vi "Free_dynamics_test.vi"() -> ()   [LabVIEW 2018]
uses:
  <vilib>/Analysis/coordinate.llb/Euler Rotation Order.ctl
  <vilib>/imath/engines/lvmath2/RunTimeEngine/NodeEndStatement/NIMS_NodeEndStatement_Output.vi
  <instcachedir>/0/NIMS_NodeEndStatement_Output_53EC0D466D134D7ABD903AC30B43404B.lvgen/NIMS_NodeEndStatement_Output_53EC0D466D134D7ABD903AC30B43404B_009.vi
  <vilib>/imath/engines/lvmath2/RunTimeEngine/ErrorHandling/NIMS_Finalize Error.vi
  <instcachedir>/0/NIMS_NodeEndStatement_Output_53EC0D466D134D7ABD903AC30B43404B.lvgen/NIMS_NodeEndStatement_Output_53EC0D466D134D7ABD903AC30B43404B_004.vi
  <vilib>/Analysis/baseanly.llb/Real Inverse Matrix.vi
  <vilib>/Analysis/Matrix/Numeric/Conversions/Array To Matrix - RA.vi
  <vilib>/Analysis/Matrix/Numeric/Conversions/Matrix To Array - RM.vi
  <vilib>/imath/engines/lvmath2/RunTimeEngine/IndexRead/NIMS M(S).vi
  <instcachedir>/0/NIMS M(S)_B826C018497E4940AE96BD27B540B6FB.lvgen/NIMS M(S)_B826C018497E4940AE96BD27B540B6FB_000.vi
  <vilib>/imathl/engines/lvmath/Functions/Error Handling/Create Error.vi
  <vilib>/imath/engines/lvmath2/RunTimeEngine/IndexRead/NIMS V(S).vi
  <instcachedir>/0/NIMS V(S)_0488751826AF41519A22953C041130DC.lvgen/NIMS V(S)_0488751826AF41519A22953C041130DC_000.vi
  <vilib>/imath/engines/lvmath2/RunTimeEngine/BuiltInFunctions/cross/NIMS_cross(GV,GV).vi
  <instcachedir>/0/NIMS_cross(GV,GV)_8E551EB9DC304C30866B49598818C259.lvgen/NIMS_cross(GV,GV)_8E551EB9DC304C30866B49598818C259_000.vi
  <vilib>/imath/engines/lvmath2/RunTimeEngine/BuiltInFunctions/double/NIMS_double.vi
  <instcachedir>/0/NIMS_double_34E32F64C2B04A25A042F4CA881A0A41.lvgen/NIMS_double_34E32F64C2B04A25A042F4CA881A0A41_002.vi
  <vilib>/imath/engines/lvmath2/RunTimeEngine/ArithmeticOperatorToken/NIMS_ArithmeticOperator_multmx.vi
  <instcachedir>/0/NIMS_ArithmeticOperator_multmx_622CA76F9646436AB036D42A9A1CE0E6.lvgen/NIMS_ArithmeticOperator_multmx_622CA76F9646436AB036D42A9A1CE0E6_004.vi
  <vilib>/imath/engines/lvmath2/RunTimeEngine/BuiltInFunctions/cross/NIMS_cross(GM,GM,I32).vi
  <instcachedir>/0/NIMS_cross(GM,GM,I32)_0F6D45CF7D834A0BB6695B819A7F63BC.lvgen/NIMS_cross(GM,GM,I32)_0F6D45CF7D834A0BB6695B819A7F63BC_000.vi
  <vilib>/imath/engines/lvmath2/RunTimeEngine/ArithmeticOperatorToken/NIMS_ArithmeticOperator_plus.vi
  <instcachedir>/0/NIMS_ArithmeticOperator_plus_DE670E32103C4C10ADF2A97367172B30.lvgen/NIMS_ArithmeticOperator_plus_DE670E32103C4C10ADF2A97367172B30_003.vi
  <vilib>/imath/engines/lvmath2/RunTimeEngine/ErrorHandling/NIMS_Create Error From Enums.vi
  <instcachedir>/0/NIMS_double_34E32F64C2B04A25A042F4CA881A0A41.lvgen/NIMS_double_34E32F64C2B04A25A042F4CA881A0A41_003.vi
  <vilib>/imath/engines/lvmath2/RunTimeEngine/ArithmeticOperatorToken/NIMS_ArithmeticOperator_multmx-internal.vi
  <instcachedir>/0/NIMS_ArithmeticOperator_multmx-internal_16A6E1DA326644AB974D30232E729C42.lvgen/NIMS_ArithmeticOperator_multmx-internal_16A6E1DA326644AB974D30232E729C42_004.vi
  <vilib>/imath/engines/lvmath2/RunTimeEngine/NodeEndStatement/NIMS_NodeEndStatement_Get Vector.vi
  <instcachedir>/0/NIMS_NodeEndStatement_Get Vector_329D0992E87F49F089135171B7FC9327.lvgen/NIMS_NodeEndStatement_Get Vector_329D0992E87F49F089135171B7FC9327_001.vi
  <vilib>/imath/engines/lvmath/Functions/Error Handling/MergeErrorsWrapper.vi
  <instcachedir>/0/NIMS_NodeEndStatement_Output_53EC0D466D134D7ABD903AC30B43404B.lvgen/NIMS_NodeEndStatement_Output_53EC0D466D134D7ABD903AC30B43404B_002.vi
  <instcachedir>/0/NIMS_NodeEndStatement_Output_53EC0D466D134D7ABD903AC30B43404B.lvgen/NIMS_NodeEndStatement_Output_53EC0D466D134D7ABD903AC30B43404B_005.vi
  <vilib>/Analysis/NI_AALPro.lvlib
  <vilib>/Analysis/Matrix/NI_Matrix.lvlib
  <vilib>/Analysis/NI_AALBase.lvlib
panel:
  out "W":dbl[](array[numeric])
  out "Yaw 2":dbl(graph)
  out "Pitch 2":dbl(graph)
  out "Roll 2":dbl(graph)
  out "Attitude 2":cluster{"phi":dbl, "theta":dbl, "psi":dbl}
  in  "Mass (kg)":dbl
  in  "MOI(kg*m^2)":dbl[][](array[numeric])
  in  "COG(m)":dbl[](array[numeric])
  in  "Simulation Time(sec)":dbl
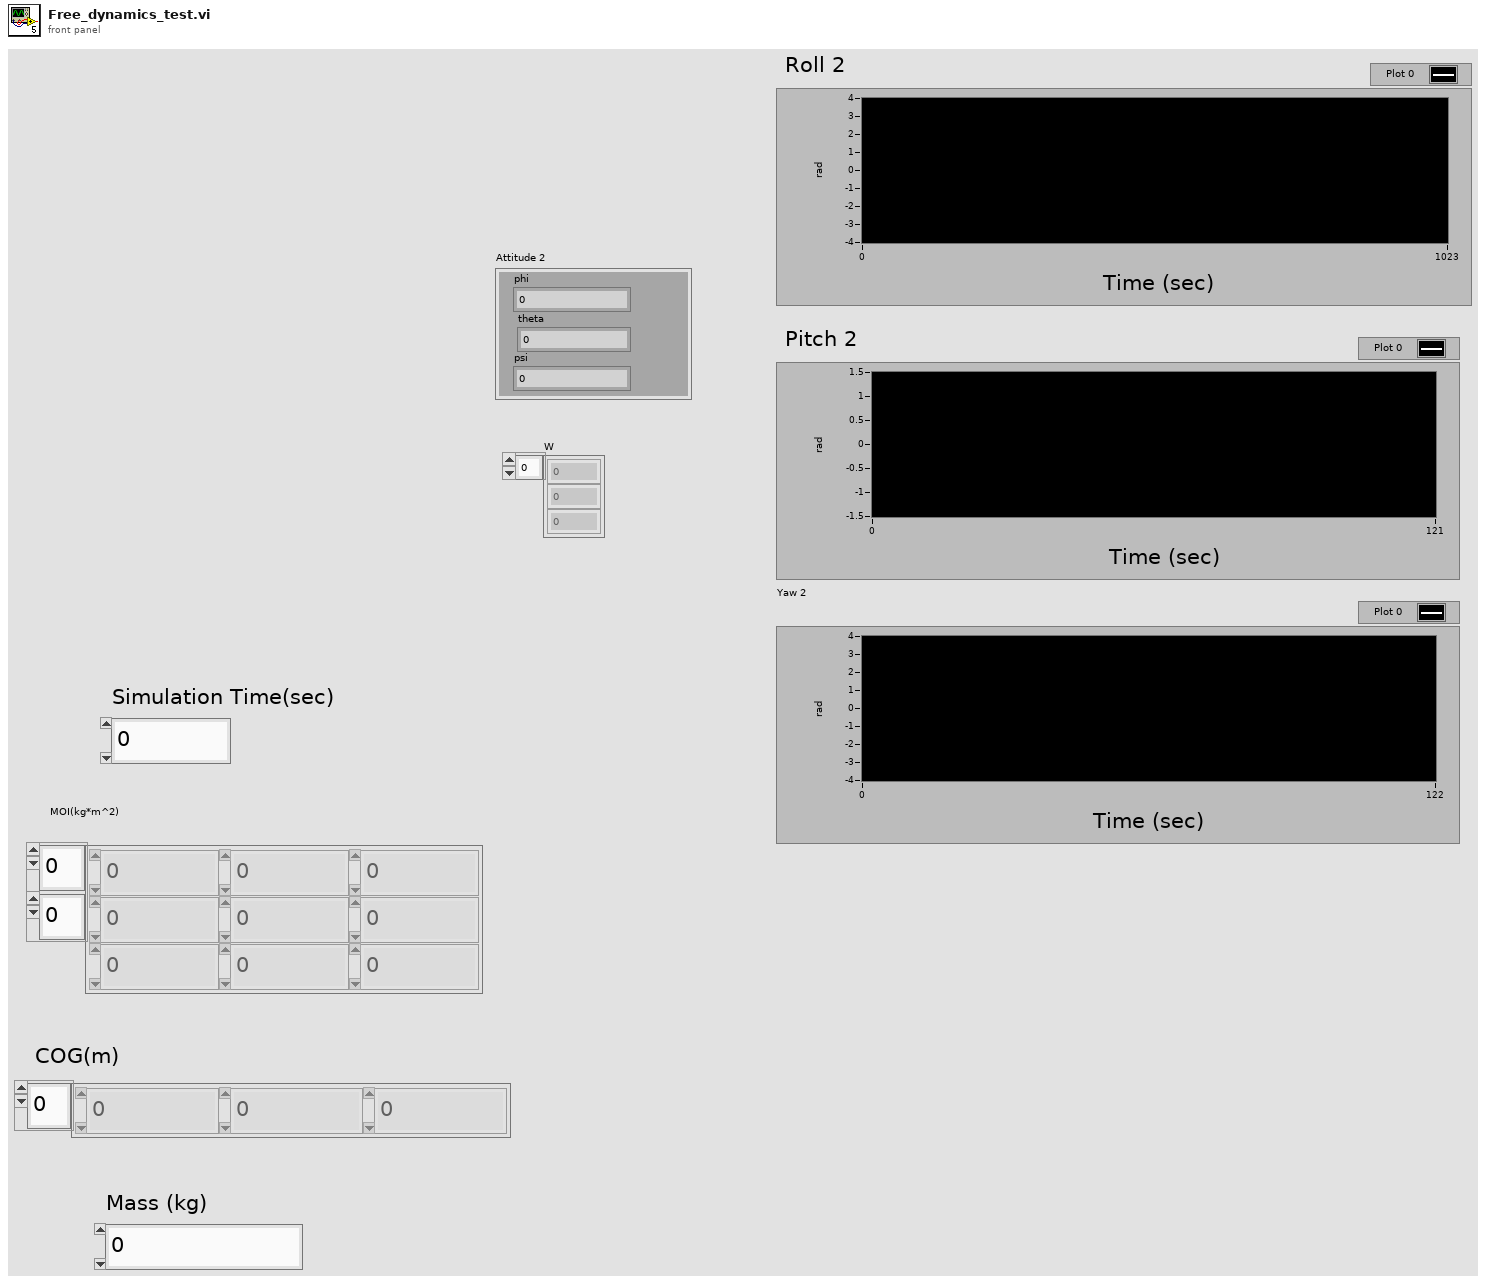
[diagram p1: front panel]
types:
  T1 = typedef "NI_AALPro.lvlib/Euler Rotation Order.ctl" = u16
  T2 = typedef "NI_Matrix.lvlib/RealMatrix.ctl" = dbl[][]
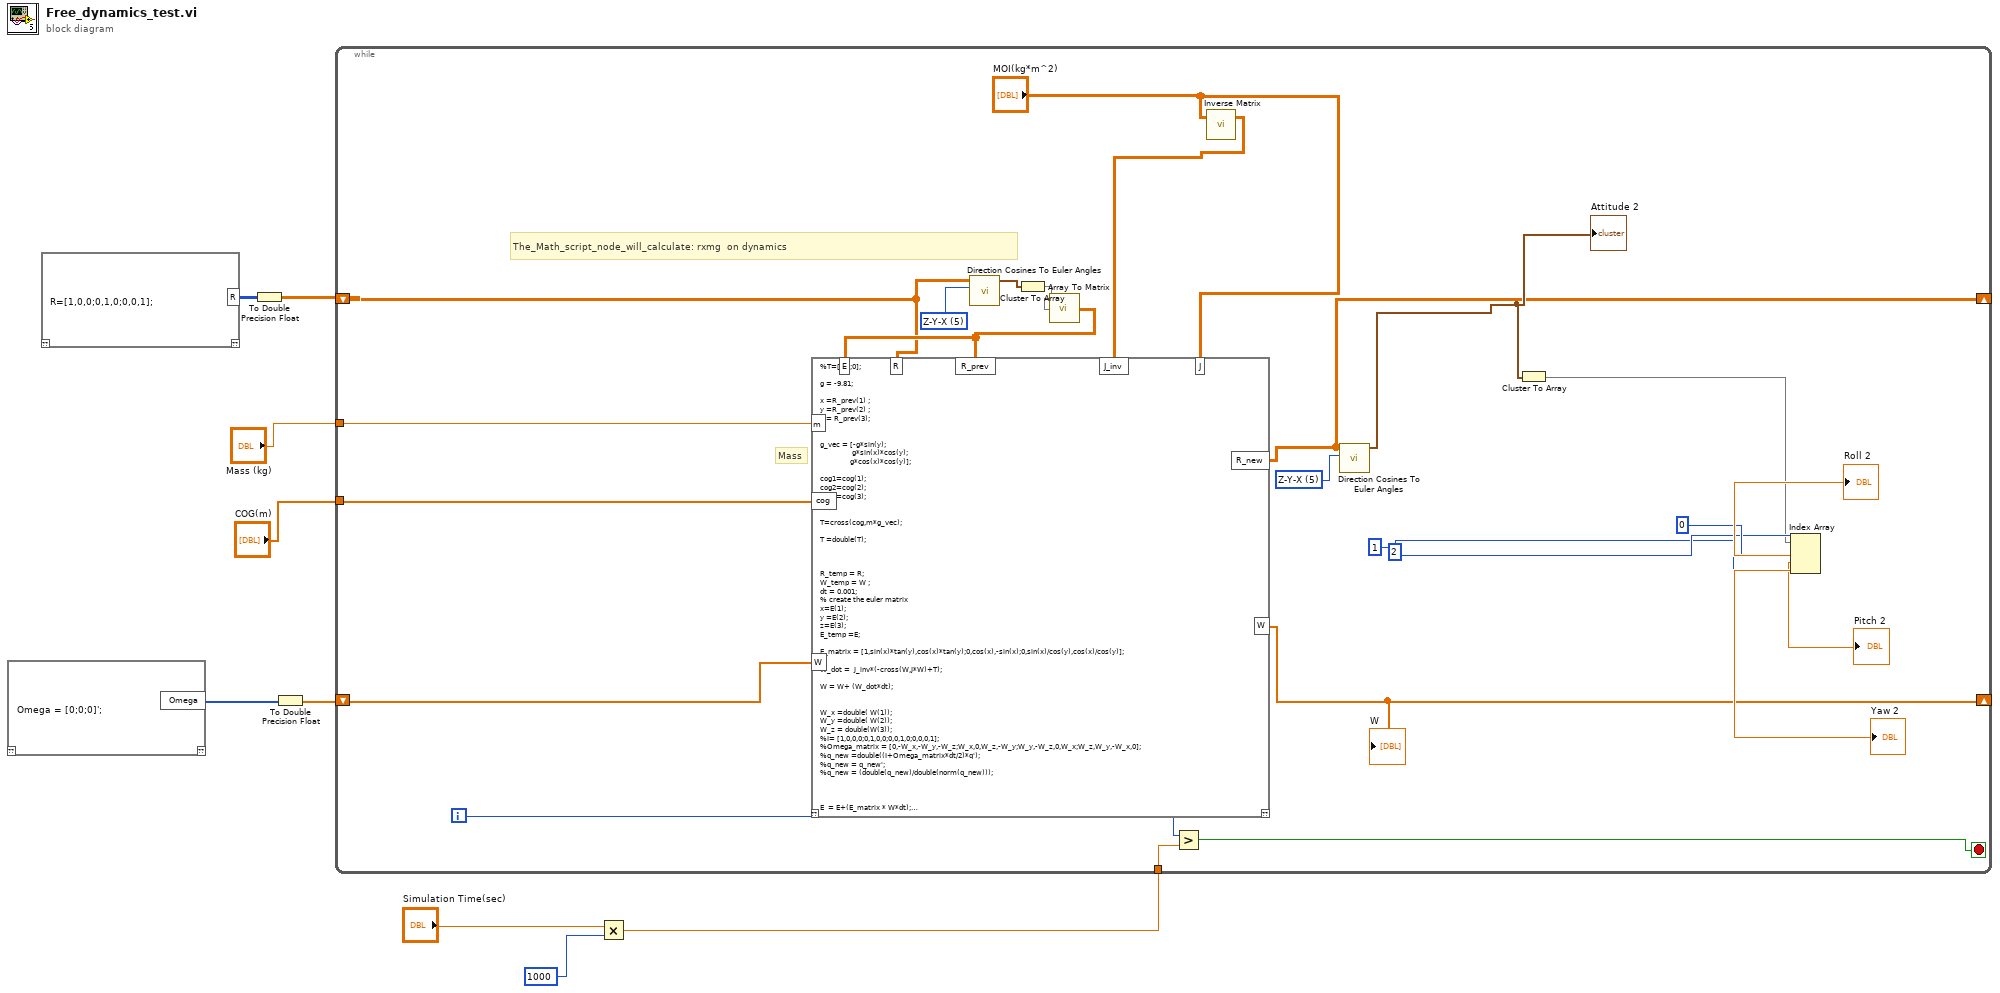
[diagram p0: block diagram]
diagram:
  # "The_Math_script_node_will_calculate: rxmg  on dynamics"
  n1 = mathscript code="Omega = [0;0;0]';"() -> ("Omega"=w6:i32[])  [unwired: 1 in, 1 out]
  n2 = mathscript code="R=[1,0,0;0,1,0;0,0,1];"() -> ("R"=w9:i32[][])  [unwired: 1 in, 1 out]
  n3 = To Double Precision Float(number=w9) -> (double precision float=w8:dbl[][])
  n4 = To Double Precision Float(number=w6) -> (double precision float=w7:dbl[])
  n5 = Multiply(x="Simulation Time(sec)", y=1000) -> (x*y=w3:dbl)
  n6 = while {
    shift-right: [w11] -> _
    shift-left: w8 -> [w17]
    shift-right: [w10] -> _
    shift-left: w7 -> [w20]
    tunnel: w3 -> [w33]
    tunnel: "Mass (kg)" -> [w19]
    tunnel: "COG(m)" -> [w18]
    i -> [w32]
    stop <- w31 stop-if-true
    w14 = T1 5 items=["X-Y-Z", "X-Z-Y", "Y-X-Z", "Y-Z-X", "Z-X-Y", "Z-Y-X", "X-Y-X", "X-Z-X", "Y-X-Y", "Y-Z-Y", "Z-X-Z", "Z-Y-Z"] ("rotation order")
    w28 = T1 5 items=["X-Y-Z", "X-Z-Y", "Y-X-Z", "Y-Z-X", "Z-X-Y", "Z-Y-X", "X-Y-X", "X-Z-X", "Y-X-Y", "Y-Z-Y", "Z-X-Z", "Z-Y-Z"] ("rotation order")
    # "Mass"
    n7 = call <vilib>:"Direction Cosines To Euler Angles.vi"("rotation order"=w28, "Direction Cosines"=w17) -> ("Euler Angles"=w30:cluster{"phi":dbl, "theta":dbl, "psi":dbl})  [unwired: 8 in, 1 out]
    n8 = Cluster To Array(cluster=w30) -> (array=w29:dbl[])
    n9 = call-poly <vilib>:"Array To Matrix.vi"("Real 1D Array"=w29) -> ("Real Matrix (Column Vector)"=w27:T2)
    n10 = Greater?(x=w32, y=w33) -> (0:w31:bool)
    n11 = call-poly <vilib>:"Inverse Matrix.vi"("Input Matrix"="MOI(kg*m^2)") -> ("Inverse Matrix"=w16:T2)  [unwired: 1 in, 1 out]
    n12 = mathscript code="%T=[0;0;0];\n\ng = -9.81;\n\nx =R_prev(1) ;\ny =R_prev(2) ;\nz = R_prev(3);\n\n\ng_vec = [-g*sin(y);\n                g*sin(x)*cos(y);\n               g*cos(x)*cos(y)];\n\ncog1=cog(1);\ncog2=cog(2);\ncog3=cog(3);\n\n\nT=cross(cog,m*g_vec);\n\nT =double(T);\n\n\n\nR_temp = R;\nW_temp = W ;\ndt = 0.001;\n% create the euler matrix\nx=E(1);\ny =E(2);\nz=E(3);\nE_temp =E;\n\nE_matrix = [1,sin(x)*tan(y),cos(x)*tan(y);0,cos(x),-sin(x);0,sin(x)/cos(y),cos(x)/cos(y)];\n\nW_dot =  J_inv*(-cross(W,J*W)+T);\n\nW = W+ (W_dot*dt);\n\n\nW_x =double( W(1));\nW_y =double( W(2));\nW_z = double(W(3));\n%I= [1,0,0,0;0,1,0,0;0,0,1,0;0,0,0,1];\n%Omega_matrix = [0,-W_x,-W_y,-W_z;W_x,0,W_z,-W_y;W_y,-W_z,0,W_x;W_z,W_y,-W_x,0];\n%q_new =double((I+Omega_matrix*dt/2)*q');\n%q_new = q_new';\n%q_new = (double(q_new)/double(norm(q_new)));\n\n\n\nE  = E+(E_matrix * W*dt);\nx = E(1);\ny = E(2);\nz = E(3);\nRx=[1,0,0;0,cos(x),-sin(x);0,sin(x),cos(x)];\nRy=[cos(y),0,sin(y);0,1,0;-sin(y),0,cos(y)];\nRz =[cos(z),-sin(z),0;sin(z),cos(z),0;0,0,1];\n\nR_new =Rz*Ry*Rx;"("m"=w19, "cog"=w18, "R_prev"=w27, "J_inv"=w16, "J"="MOI(kg*m^2)", "R"=w17, "W"=w20, "E"=w27) -> ("W"=w10:dbl[], "R_new"=w11:dbl[][])  [unwired: 1 in, 1 out]
    "W" <- w10
    n13 = call <vilib>:"Direction Cosines To Euler Angles.vi"("rotation order"=w14, "Direction Cosines"=w11) -> ("Euler Angles"=w13:cluster{"phi":dbl, "theta":dbl, "psi":dbl})  [unwired: 8 in, 1 out]
    "Attitude 2" <- w13
    n14 = Cluster To Array(cluster=w13) -> (array=w12:dbl[])
    n15 = Index Array(array=w12, index #1=0 ("index"), index #2=1 ("index"), index #3=2 ("index")) -> (element #1=→"Roll 2":dbl, element #2=→"Pitch 2":dbl, element #3=→"Yaw 2":dbl)
  }
